vi "Test Tiff.vi"(8 "error in (no error)":errorcluster, 10 "message":string, 11 "Tiff Writer in":refnum<class "Tiff Writer.lvclass">) -> (0 "error out":errorcluster, 3 "Tiff Writer out":refnum<class "Tiff Writer.lvclass">)   [LabVIEW 2018]
uses:
  Tiff Writer.lvclass
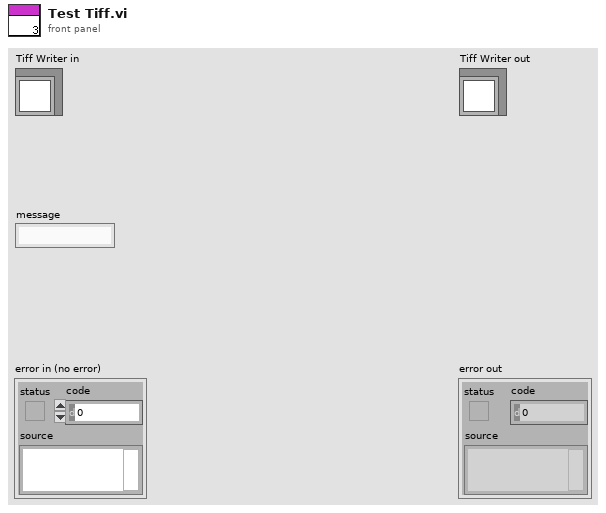
[diagram p1: front panel]
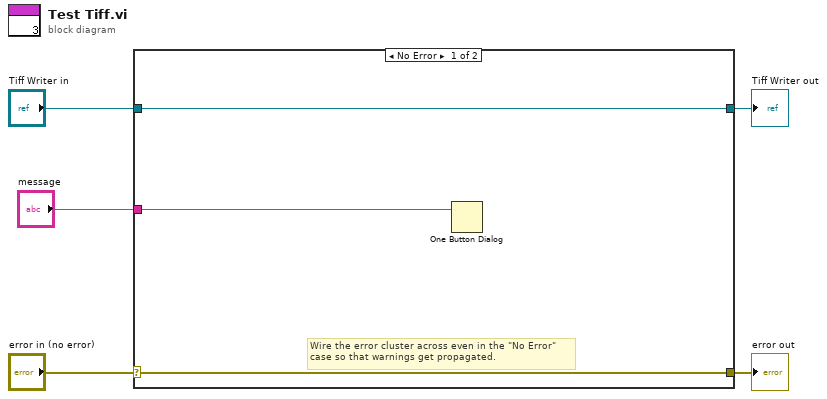
[diagram p0: block diagram]
diagram:
  n1 = case shown="No Error" "error in (no error)" {
    selector: "error in (no error)" -> [w7 w10]
    tunnel: [w7 w10] -> w4
    tunnel: [w8 w9] -> w2
    tunnel: "Tiff Writer in" -> [w8 w9]
    tunnel: "message" -> [w6 _]
    frame No Error {
      # "Wire the error cluster across even in the \"No Error\"\ncase so that warnings get propagated."
      n2 = One Button Dialog(message=w6) -> ()  [unwired: 1 in, 1 out]
    }
    frame Error {
    }
  }
  "error out" <- w4
  "Tiff Writer out" <- w2
